vi "FlagToRing.vi"() -> ()   [LabVIEW 2024]
uses:
  <vilib>/regexp/Match Regular Expression.xnode
panel:
  in  "flags (0)":u32(ring) items=["0"=0, "SDL_WINDOW_FULLSCREEN"=1, "SDL_WINDOW_OPENGL"=2, "SDL_WINDOW_OCCLUDED"=4, "SDL_WINDOW_HIDDEN"=8, "SDL_WINDOW_BORDERLESS"=16, "SDL_WINDOW_RESIZABLE"=32, "SDL_WINDOW_MINIMIZED"=64, "SDL_WINDOW_MAXIMIZED"=128, "SDL_WINDOW_MOUSE_GRABBED"=256, "SDL_WINDOW_INPUT_FOCUS"=512, "SDL_WINDOW_MOUSE_FOCUS"=1024, "SDL_WINDOW_EXTERNAL"=2048, "SDL_WINDOW_MODAL"=4096, "SDL_WINDOW_HIGH_PIXEL_DENSITY"=8192, "SDL_WINDOW_MOUSE_CAPTURE"=16384, "SDL_WINDOW_MOUSE_RELATIVE_MODE"=32768, "SDL_WINDOW_ALWAYS_ON_TOP"=65536, "SDL_WINDOW_UTILITY"=131072, "SDL_WINDOW_TOOLTIP"=262144, "SDL_WINDOW_POPUP_MENU"=524288, "SDL_WINDOW_KEYBOARD_GRABBED"=1048576, "SDL_WINDOW_VULKAN"=268435456, "SDL_WINDOW_METAL"=536870912, "SDL_WINDOW_TRANSPARENT"=1073741824, "SDL_WINDOW_NOT_FOCUSABLE"=2147483648]
  in  "#Define list":string="#define SDL_WINDOW_FULLSCREEN           SDL_UINT64_C(0x0000000000000001)    /**< window is in fullscreen mode */\n#define SDL_WINDOW_OPENGL               SDL_UINT64_C(0x0000000000000002)    /**< window usable with OpenGL context */\n#define SDL_WINDOW_OCCLUDED             SDL_UINT64_C(0x0000000000000004)    /**< window is occluded */\n#define SDL_WINDOW_HIDDEN               SDL_UINT64_C(0x0000000000000008)    /**< window is neither mapped onto the desktop nor shown in the taskbar/dock/window list; SDL_ShowWindow() is required for it to become visible */\n#define SDL_WINDOW_BORDERLESS           SDL_UINT64_C(0x0000000000000010)    /**< no window decoration */\n#define SDL_WINDOW_RESIZABLE            SDL_UINT64_C(0x0000000000000020)    /**< window can be resized */\n#define SDL_WINDOW_MINIMIZED            SDL_UINT64_C(0x0000000000000040)    /**< window is minimized */\n#define SDL_WINDOW_MAXIMIZED            SDL_UINT64_C(0x0000000000000080)    /**< window is maximized */\n#define SDL_WINDOW_MOUSE_GRABBED        SDL_UINT64_C(0x0000000000000100)    /**< window has grabbed mouse input */\n#define SDL_WINDOW_INPUT_FOCUS          SDL_UINT64_C(0x0000000000000200)    /**< window has input focus */\n#define SDL_WINDOW_MOUSE_FOCUS          SDL_UINT64_C(0x0000000000000400)    /**< window has mouse focus */\n#define SDL_WINDOW_EXTERNAL             SDL_UINT64_C(0x0000000000000800)    /**< window not created by SDL */\n#define SDL_WINDOW_MODAL                SDL_UINT64_C(0x0000000000001000)    /**< window is modal */\n#define SDL_WINDOW_HIGH_PIXEL_DENSITY   SDL_UINT64_C(0x0000000000002000)    /**< window uses high pixel density back buffer if possible */\n#define SDL_WINDOW_MOUSE_CAPTURE        SDL_UINT64_C(0x0000000000004000)    /**< window has mouse captured (unrelated to MOUSE_GRABBED) */\n#define SDL_WINDOW_MOUSE_RELATIVE_MODE  SDL_UINT64_C(0x0000000000008000)    /**< window has relative mode enabled */\n#define SDL_WINDOW_ALWAYS_ON_TOP        SDL_UINT64_C(0x0000000000010000)    /**< window should always be above others */\n#define SDL_WINDOW_UTILITY              SDL_UINT64_C(0x0000000000020000)    /**< window should be treated as a utility window, not showing in the task bar and window list */\n#define SDL_WINDOW_TOOLTIP              SDL_UINT64_C(0x0000000000040000)    /**< window should be treated as a tooltip and does not get mouse or keyboard focus, requires a parent window */\n#define SDL_WINDOW_POPUP_MENU           SDL_UINT64_C(0x0000000000080000)    /**< window should be treated as a popup menu, requires a parent window */\n#define SDL_WINDOW_KEYBOARD_GRABBED     SDL_UINT64_C(0x0000000000100000)    /**< window has grabbed keyboard input */\n#define SDL_WINDOW_VULKAN               SDL_UINT64_C(0x0000000010000000)    /**< window usable for Vulkan surface */\n#define SDL_WINDOW_METAL                SDL_UINT64_C(0x0000000020000000)    /**< window usable for Metal view */\n#define SDL_WINDOW_TRANSPARENT          SDL_UINT64_C(0x0000000040000000)    /**< window with transparent buffer */\n#define SDL_WINDOW_NOT_FOCUSABLE        SDL_UINT64_C(0x0000000080000000)    /**< window should not be focusable */"
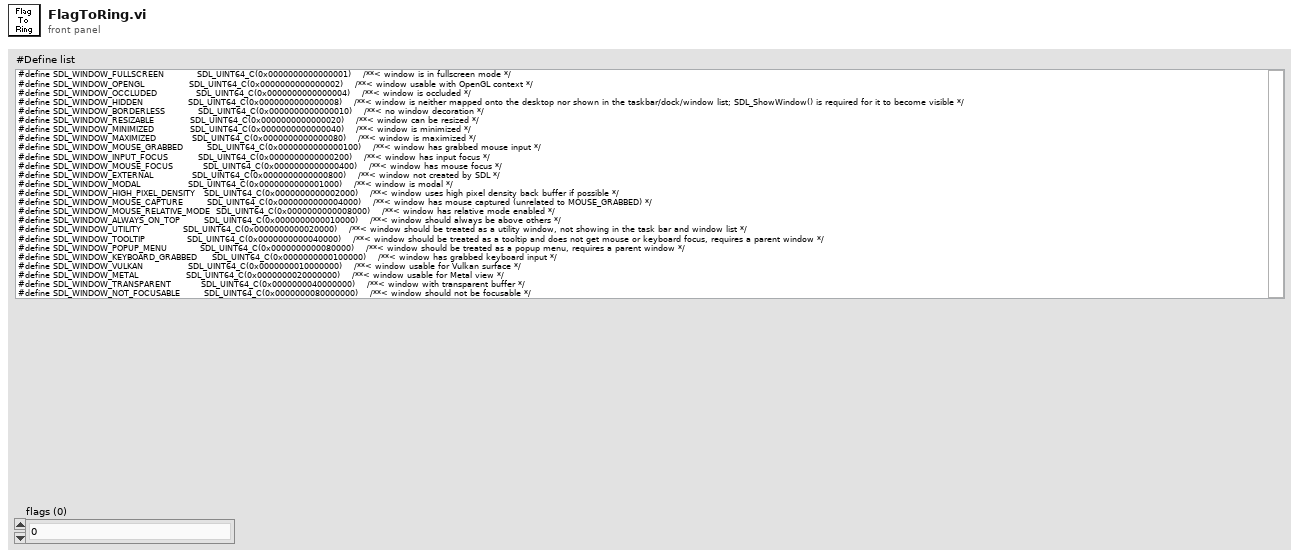
[diagram p1: front panel]
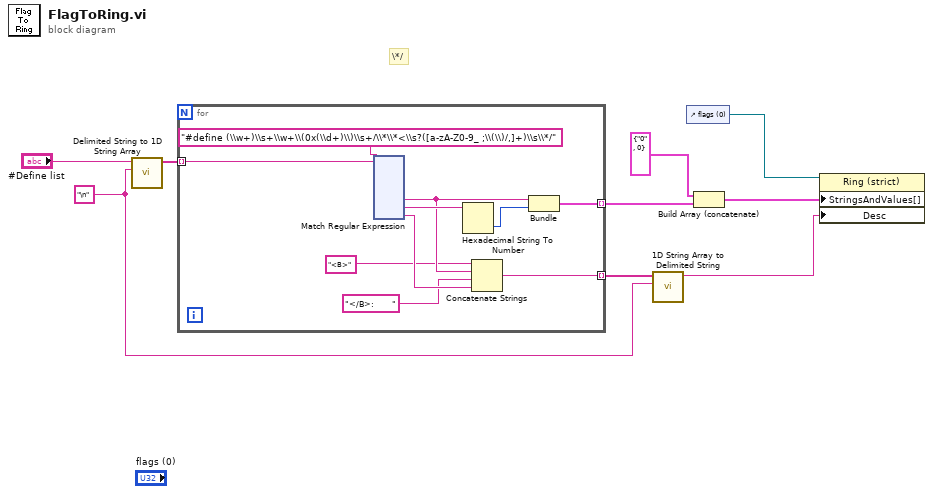
[diagram p0: block diagram]
diagram:
  w5 = "\n" ("delimiter")
  # "\\*/"
  n1 = call <vilib>:"Delimited String to 1D String Array.vi"("delimiter"=w5, "delimited string"="#Define list") -> ("string array"=w8:string[])  [unwired: 9 in]
  n2 = for {
    tunnel: w8 -> [w19] mode=indexing
    tunnel: [w16] -> w7 mode=indexing
    tunnel: [w12] -> w6 mode=indexing
    n3 = xnode "Match Regular Expression"("input string"=w19, "regular expression"="#define (\\w+)\\s+\\w+\\(0x(\\d+)\\)\\s+/\\*\\*<\\s?([a-zA-Z0-9_ ;\\(\\)/,]+)\\s\\*/") -> ("submatch 1"=w14:string, "submatch 2"=w17:string, "submatch 3"=w13:string)  [unwired: 4 in, 5 out]
    n4 = Hexadecimal String To Number(string=w17) -> (number=w15:u32)  [unwired: 2 in, 1 out]
    n5 = Concatenate Strings("<B>" ("string"), w14, "</B>:      " ("string"), w13) -> (w12:string)
    n6 = Bundle("submatch 1"=w14, w15) -> (w16:cluster{"submatch 1":string, u32})  [unwired: 1 in]
  }
  n7 = call <vilib>:"1D String Array to Delimited String.vi"("delimiter"=w5, "string array"=w6) -> ("delimited string"=w1:string)  [unwired: 9 in]
  n8 = control-ref of="flags (0)"() -> (w4:refnum<vi>)
  n9 = Build Array (concatenate)(cluster{"submatch 1":string, u32} {"submatch 1"="0", 0}, w7) -> (w3:cluster{"submatch 1":string, u32}[])
  n10 = property class="Ring (strict)"(reference=w4, "StringsAndValues[]"=w3, "Desc"=w1) -> ()  [unwired: 1 in, 2 out]
